vi "_unittest Reshape Array.vi"(10 "Sizes":i32[](array[numeric]), 11 "Array Elements":string[](array[string])) -> (3 "String":string)   [LabVIEW 2018, in "labview_json_tests.lvlib"]
uses:
  labview_json_tests.lvlib
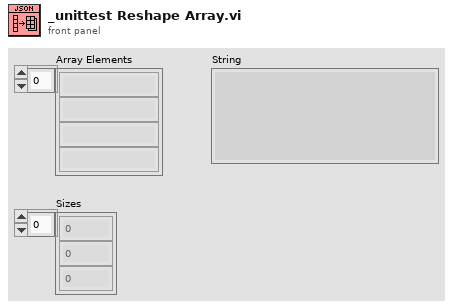
[diagram p1: front panel]
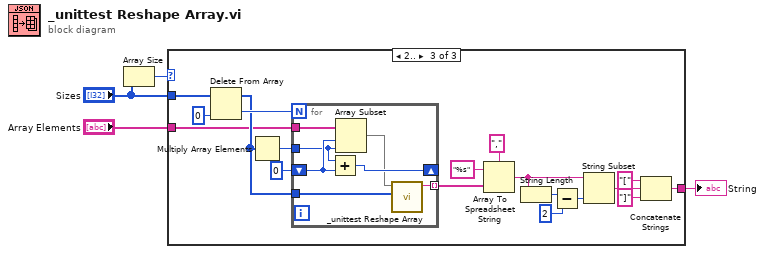
[diagram p0: block diagram]
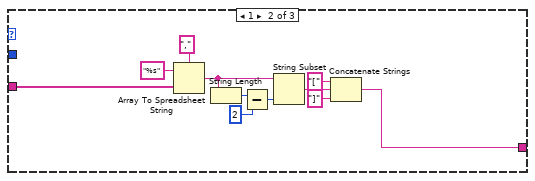
[diagram p3: hidden frame]
diagram:
  n1 = Array Size(array="Sizes") -> (size(s)=w1:i32)
  n2 = case shown="2.." w1 {
    tunnel: "Array Elements" -> [_ w6 w28]
    tunnel: "Sizes" -> [_ _ w27]
    tunnel: [_ w5 w16] -> w3
    frame ..0 {
    }
    frame 1 {
      n3 = Array To Spreadsheet String(delimiter (Tab)=",", array=w6, 3:"%s" ("format string")) -> (spreadsheet string=w9:string)
      n4 = String Length(string=w9) -> (length=w10:i32)
      n5 = Subtract(x=w10, y=2) -> (x-y=w12:i32)
      n6 = String Subset(string=w9, length (rest)=w12) -> (substring=w13:string)  [unwired: 1 in]
      n7 = Concatenate Strings("[" ("string"), w13, "]" ("string")) -> (w5:string)
    }
    frame 2.. {
      n8 = Delete From Array(array=w27, index=0) -> (deleted portion=w30:i32, array with subset deleted=w29:i32[])  [unwired: 1 in]
      n9 = Multiply Array Elements(1:w29) -> (0:w31:i32)
      n10 = for {
        N: w30 -> [_]
        tunnel: w28 -> [w40]
        shift-right: [w37] -> _
        shift-left: 0 -> [w39]
        tunnel: w31 -> [w38]
        tunnel: w29 -> [w36]
        tunnel: [w34] -> w17 mode=indexing
        n11 = Add(x=w38, y=w39) -> (x+y=w37:i32)
        n12 = Array Subset(array=w40, index=w39, length=w38) -> (w35:string[])
        n13 = call "_unittest Reshape Array.vi"("Sizes"=w36, "Array Elements"=w35) -> ("String"=w34:string)  [unwired: 9 in]
      }
      n14 = Array To Spreadsheet String(delimiter (Tab)=",", array=w17, 3:"%s" ("format string")) -> (spreadsheet string=w20:string)
      n15 = String Length(string=w20) -> (length=w21:i32)
      n16 = Subtract(x=w21, y=2) -> (x-y=w23:i32)
      n17 = String Subset(string=w20, length (rest)=w23) -> (substring=w24:string)  [unwired: 1 in]
      n18 = Concatenate Strings("[" ("string"), w24, "]" ("string")) -> (w16:string)
    }
  }
  "String" <- w3
